vi "read_delimiter.vi"() -> ()   [LabVIEW 2022 SP3]
uses:
  <vilib>/Utility/file.llb/Read Delimited Spreadsheet (I64).vi
panel:
  out "all rows":i64[][](array[numeric])
  in  "file path (dialog if empty)":path
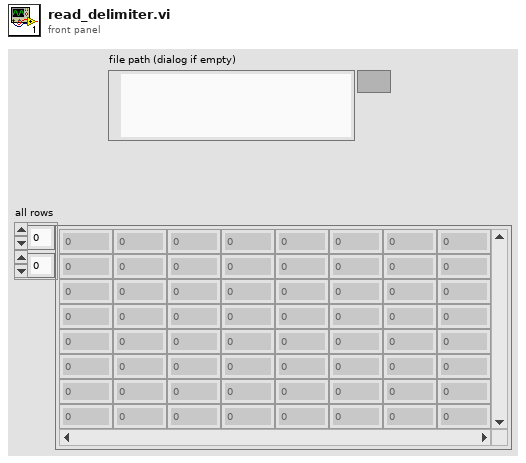
[diagram p1: front panel]
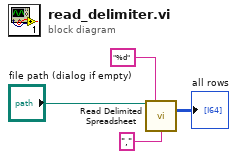
[diagram p0: block diagram]
diagram:
  n1 = call-poly <vilib>:"Read Delimited Spreadsheet.vi"("file path (dialog if empty)"="file path (dialog if empty)", "format (%d)"="%d" ("format (%s)"), "delimiter (\\t)"="," ("delimiter (\\t)")) -> ("all rows"=→"all rows":i64[][])  [unwired: 7 in, 5 out]
